vi "down_cast.vi"(8 "error in (no error)":errorcluster, 11 "GenericTrajectory.lvclass":refnum<class "GenericTrajectory.lvclass">) -> (0 "error out":errorcluster, 3 "TrajectoryDL091126GenericVoxel out":refnum<class "TrajectoryDL091126GenericVoxel.lvclass">)   [LabVIEW 2010, in "TrajectoryDL091126GenericVoxel.lvclass"]
uses:
  TrajectoryDL091126GenericVoxel.lvclass
  GenericTrajectory/GenericTrajectory/GenericTrajectory.lvclass
  common/classes/ErrorController/ErrorController/class_data.vi
  common/classes/ErrorController/ErrorController/ErrorController.lvclass
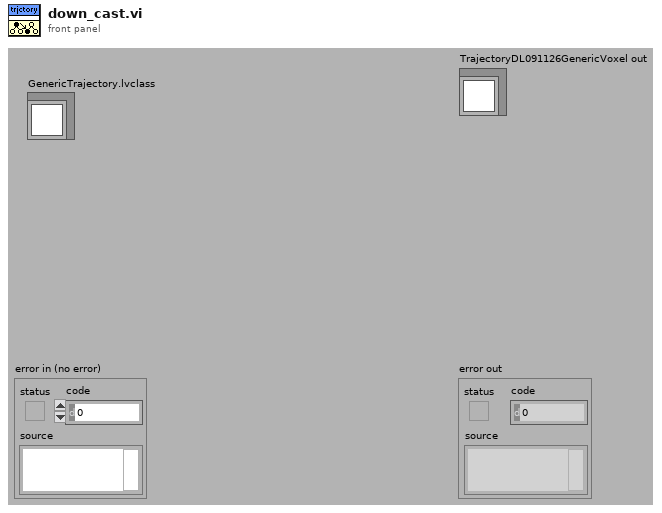
[diagram p1: front panel]
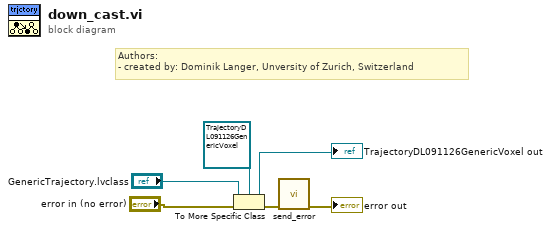
[diagram p0: block diagram]
diagram:
  # "Authors: \n- created by: Dominik Langer, Unversity of Zurich, Switzerland"
  n1 = To More Specific Class(target class=refnum<class "TrajectoryDL091126GenericVoxel.lvclass"> refnum ("TrajectoryDL091126GenericVoxel.lvclass"), reference="GenericTrajectory.lvclass", error in="error in (no error)") -> (specific class reference=→"TrajectoryDL091126GenericVoxel out":refnum<class "TrajectoryDL091126GenericVoxel.lvclass">, error out=w2:errorcluster)
  n2 = call "send_error.vi"("error in (no error)"=w2) -> ("error out"=→"error out":errorcluster)  [unwired: 10 in]
